vi "Make initial guess (N.O.).vi"(6 "Positive?":bool, 7 "input cluster":T1, 8 "error in (no error)":errorcluster, 9 "Desired Field":dbl, 10 "Voltage Limit":dbl=2255.0 format="%.2f", 11 "VISA session":refnum<visa-resource-name>) -> (0 "error out":errorcluster, 2 "Current guess":dbl, 3 "dup VISA session":refnum<visa-resource-name>, 5 "output cluster":T1)   [LabVIEW 2012]
uses:
  Magna Power Constants.vi
  <vilib>/gmath/NI_Gmath.lvlib
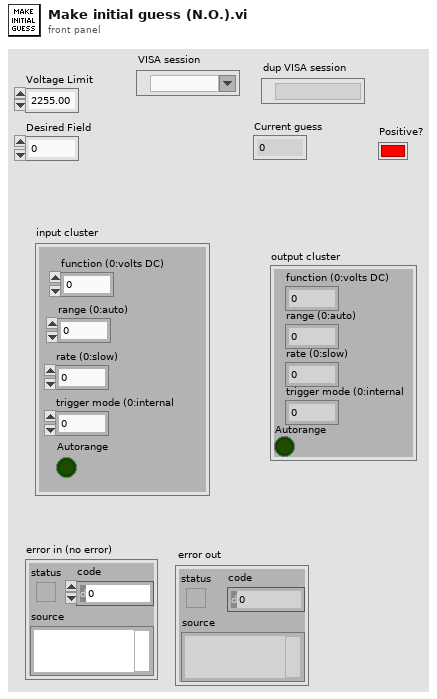
[diagram p1: front panel]
types:
  T1 = cluster{"function (0:volts DC)":i16, "range (0:auto)":i16, "rate (0:slow)":i16, "trigger mode (0:internal":i16, "Autorange":bool}
  T2 = cluster{"Magna Current":dbl[], "Magnetic Field":dbl[], "Fluke Voltage":dbl[]}
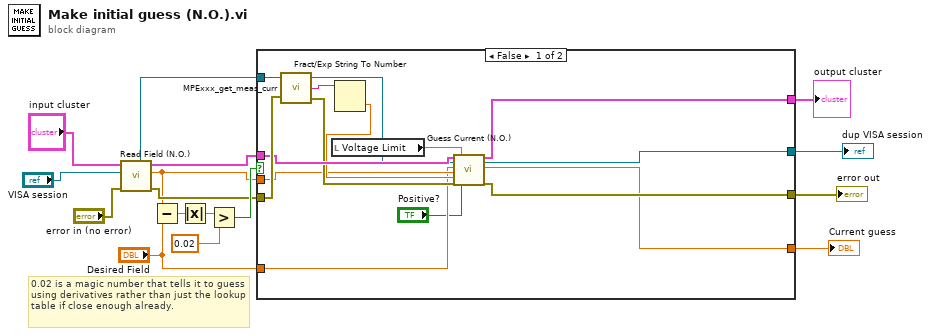
[diagram p0: block diagram]
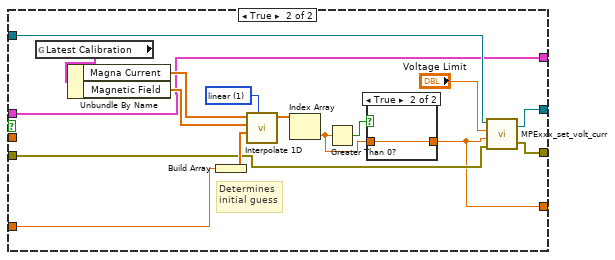
[diagram p2: hidden frame]
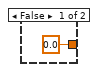
[diagram p3: hidden frame]
diagram:
  # "0.02 is a magic number that tells it to guess using derivatives rather than just the lookup table if close enough already."
  n1 = call "Read Field (N.O.).vi"("error in (no error)"="error in (no error)", "VISA session"="VISA session", "input cluster"="input cluster") -> ("error out"=w8:errorcluster, "Field (T)"=w2:dbl, "output cluster"=w3:T1, "dup VISA session"=w9:refnum<visa-resource-name>)  [unwired: 3 in, 2 out]
  n2 = Subtract(x=w2, y="Desired Field") -> (x-y=w13:dbl)
  n3 = Absolute Value(x=w13) -> (abs(x)=w12:dbl)
  n4 = Greater?(x=w12, y=0.02) -> (0:w10:bool)
  n5 = case shown="False" w10 {
    tunnel: w9 -> [w31 w38]
    tunnel: w8 -> [w30 w37]
    tunnel: "Desired Field" -> [w22 w36]
    tunnel: [w19 w35] -> w6
    tunnel: [w18 w34] -> w5
    tunnel: [w17 w33] -> w4
    tunnel: w3 -> [w27 w32]
    tunnel: w2 -> [w23 _]
    tunnel: [w20 w32] -> w1
    frame False {
      n6 = call "MPExxx_get_meas_curr.vi"("VISA session"=w31, "error in (no error)"=w30) -> ("dup VISA session"=w26:refnum<visa-resource-name>, "Output Current"=w29:string, "error out"=w25:errorcluster)
      n7 = local read "Voltage Limit"() -> (w28:dbl)
      n8 = Fract/Exp String To Number(string=w29) -> (number=w24:dbl)  [unwired: 3 in, 1 out]
      n9 = call "Guess Current (N.O.).vi"("input cluster"=w27, "VISA session"=w26, "Desired Field"=w22, "Actual Field old"=w23, "Current guess"=w24, "error in (no error)"=w25, "Voltage Limit"=w28, "Positive?"="Positive?") -> ("output cluster"=w20:T1, "dup VISA session"=w19:refnum<visa-resource-name>, "New guess"=w17:dbl, "error out"=w18:errorcluster)  [unwired: 7 in, 1 out]
    }
    frame True {
      w46 = 1 items=["nearest", "linear", "spline", "cubic Hermite", "Lagrange"] ("method")
      # "Determines\ninitial guess"
      n10 = global read "Magna Power Constants.vi" "Latest Calibration"() -> (w47:T2)
      n11 = Unbundle By Name(w47) -> ("Magna Current"=w42:dbl[], "Magnetic Field"=w43:dbl[])
      n12 = Build Array(w36) -> (w45:dbl[])
      n13 = call <vilib>:"Interpolate 1D.vi"("method"=w46, "xi"=w45, "X"=w43, "Y"=w42) -> ("yi"=w44:dbl[])  [unwired: 5 in, 2 out]
      n14 = Index Array(array=w44) -> (element=w39:dbl)  [unwired: 1 in]
      n15 = Greater Than 0?(x=w39) -> (x > 0?=w40:bool)
      n16 = case shown="True" w40 {
        tunnel: [0.0 ("Numeric") w49] -> w33
        tunnel: w39 -> [_ w49]
        frame False {
        }
        frame True {
        }
      }
      n17 = call "MPExxx_set_volt_curr.vi"("error in (no error)"=w37, "Set Current"=w33, "Set Voltage"="Voltage Limit", "VISA session"=w38) -> ("error out"=w34:errorcluster, "dup VISA session"=w35:refnum<visa-resource-name>)
    }
  }
  "Current guess" <- w4
  "error out" <- w5
  "dup VISA session" <- w6
  "output cluster" <- w1
